vi "Send Command.vi"(8 "error in (no error)":errorcluster, 11 "GenericGuiAO in":refnum<class "GenericGuiAO.lvclass">) -> (0 "error out":errorcluster, 3 "GenericGuiAO out":refnum<class "GenericGuiAO.lvclass">)   [LabVIEW 2023, in "VolatusDAQGenericGUI.lvlib" / "GenericGuiAO.lvclass"]
uses:
  GenericGuiAO.lvclass
  GenericGuiAO.lvclass/GenericGuiAO.ctl
  Volatus/Module/Module.lvclass
  messages/CmdAnalog/Data.ctl
  messages/CmdAnalog/CmdAnalog.lvlib
  C:/dev/volatus/mts-volatus-super/libs/lv-volatus/Volatus/Module/Module.lvclass
  C:/dev/volatus/mts-volatus-super/libs/lv-volatus/VolatusDAQGenericGUI/GenericGuiAO/GenericGuiAO.lvclass
  Volatus/VolatusAPI/VolatusAPI.lvclass
  Volatus/Module Identity/Module Identity.lvclass
  Volatus/MessageQ/MessageQ.lvclass
  messages/CmdAnalogMultiple/Class/Msg.lvclass
  messages/CmdAnalogMultiple/CmdAnalogMultiple.lvlib
  C:/dev/volatus/mts-volatus-super/libs/lv-volatus/messages/CmdAnalogMultiple/Class/Msg.lvclass
  C:/dev/volatus/mts-volatus-super/libs/lv-protoc/LV-Proto/Message/Message.lvclass
  C:/dev/volatus/mts-volatus-super/libs/lv-volatus/Volatus/Module Identity/Module Identity.lvclass
  C:/dev/volatus/mts-volatus-super/libs/lv-volatus/Volatus/Identity/Identity.lvclass
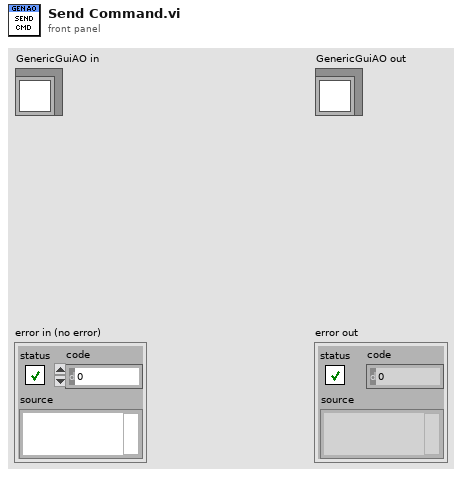
[diagram p1: front panel]
types:
  T1 = typedef "VolatusDAQGenericGUI.lvlib/Group Info.ctl" = cluster{"Group":refnum<class "Group DBL.lvclass">, "Channel Names":string[], "Resources":string[], "Node":string, "Task":string}
  T2 = typedef "CmdAnalog.lvlib/Data.ctl" = cluster{"channel":string, "value":dbl}
  T3 = typedef "CmdAnalogMultiple.lvlib/Data.ctl" = cluster{"values":T2[]}
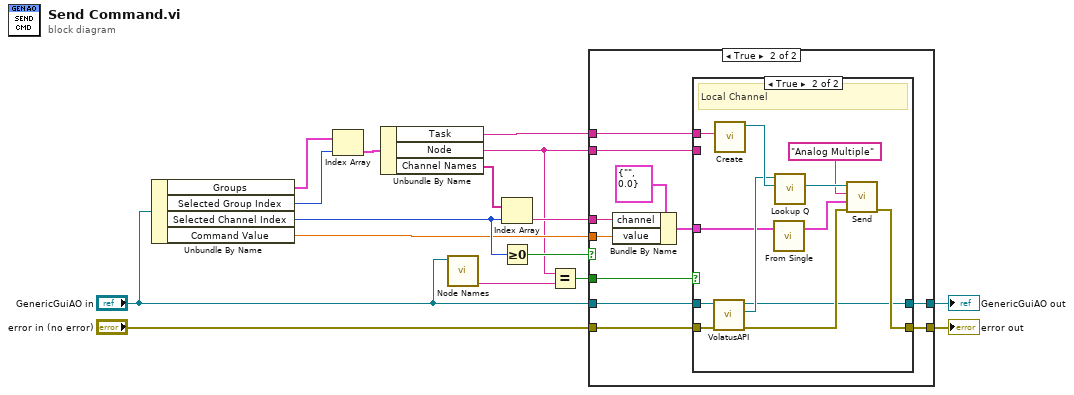
[diagram p0: block diagram]
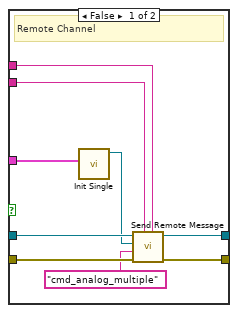
[diagram p3: hidden frame]
diagram:
  n1 = Unbundle By Name("GenericGuiAO in") -> ("Groups"=w13:T1[], "Selected Group Index"=w12:i32, "Selected Channel Index"=w9:i32, "Command Value"=w7:dbl)
  n2 = Index Array(array=w13, index=w12) -> (element=w11:T1)
  n3 = Unbundle By Name(w11) -> ("Task"=w6:string, "Node"=w4:string, "Channel Names"=w10:string[])
  n4 = call "Node Names.vi"("Module in"="GenericGuiAO in") -> ("Node"=w3:string)  [unwired: 6 in, 4 out]
  n5 = Index Array(array=w10, index=w9) -> (element=w8:string)
  n6 = Greater Or Equal To 0?(x=w9) -> (x >= 0?=w5:bool)
  n7 = Equal?(x=w4, y=w3) -> (x = y?=w1:bool)
  n8 = case shown="True" w5 {
    tunnel: "error in (no error)" -> [w17 w29]
    tunnel: [w17 w28] -> w15
    tunnel: [w18 w27] -> w14
    tunnel: "GenericGuiAO in" -> [w18 w26]
    tunnel: w8 -> [_ w25]
    tunnel: w7 -> [_ w24]
    tunnel: w4 -> [_ w23]
    tunnel: w6 -> [_ w22]
    tunnel: w1 -> [_ w19]
    frame False {
    }
    frame True {
      n9 = Bundle By Name(cluster=T2 {"channel"="", "value"=0.0} ("CmdAnalog"), "channel"=w25, "value"=w24) -> (w20:T2)
      n10 = case shown="True" w19 {
        tunnel: w29 -> [w38 w42]
        tunnel: [w37 w41] -> w28
        tunnel: [w36 w40] -> w27
        tunnel: w26 -> [w35 w47]
        tunnel: w23 -> [w34 _]
        tunnel: w22 -> [w33 w49]
        tunnel: w20 -> [w32 w43]
        frame False {
          # "Remote Channel"
          n11 = call "Init Single.vi"("value"=w32) -> ("Msg out"=w31:refnum<class "Msg.lvclass">)  [unwired: 10 in]
          n12 = call "Send Remote Message.vi"("Target Task (None)"=w33, "Target Name"=w34, "error in (no error)"=w38, "Message Type"="cmd_analog_multiple", "Message"=w31, "Module in"=w35) -> ("error out"=w37:errorcluster, "Module out"=w36:refnum<class "GenericGuiAO.lvclass">)  [unwired: 4 in]
        }
        frame True {
          # "Local Channel"
          n13 = call "VolatusAPI.vi"("Module in"=w47) -> ("VolatusAPI"=w46:refnum<class "VolatusAPI.lvclass">, "Module out"=w40:refnum<class "GenericGuiAO.lvclass">)  [unwired: 9 in]
          n14 = call "Create.vi"("ID"=w49) -> ("Module Identity out"=w48:refnum<class "Module Identity.lvclass">)  [unwired: 10 in]
          n15 = call "From Single.vi"("CmdAnalog"=w43) -> ("CmdAnalogMultiple"=w39:T3)  [unwired: 6 in]
          n16 = call "Lookup Q.vi"("Identity"=w48, "VolatusAPI in"=w46) -> ("MessageQ"=w45:refnum<class "MessageQ.lvclass">)  [unwired: 7 in, 2 out]
          n17 = call "Send.vi"("error in (no error)"=w42, "Data"=w39, "ID"="Analog Multiple", "MessageQ in"=w45) -> ("error out"=w41:errorcluster)  [unwired: 6 in, 1 out]
        }
      }
    }
  }
  "error out" <- w15
  "GenericGuiAO out" <- w14
